vi "BucleWhile.vi"() -> ()   [LabVIEW 2020]
panel:
  in  "stop":bool
  in  "Tiempo apagado":dbl
  in  "Tiempo encendido":dbl
  out "Led":bool
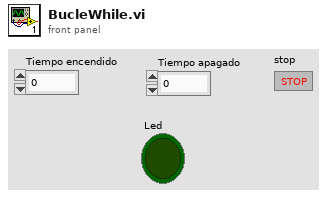
[diagram p1: front panel]
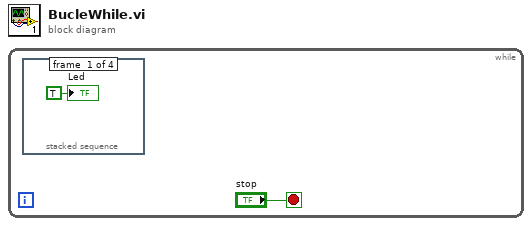
[diagram p0: block diagram]
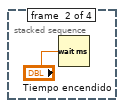
[diagram p2: hidden frame]
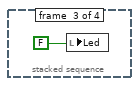
[diagram p3: hidden frame]
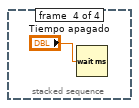
[diagram p4: hidden frame]
diagram:
  n1 = while {
    stop <- "stop" stop-if-true
    n2 = stacked-sequence {
      frame #0 {
        "Led" <- TRUE ("Led")
      }
      frame #1 {
        n3 = Wait (ms)(milliseconds to wait="Tiempo encendido") -> ()  [unwired: 1 out]
      }
      frame #2 {
        n4 = local write "Led"(FALSE ("Led")) -> ()
      }
      frame #3 {
        n5 = Wait (ms)(milliseconds to wait="Tiempo apagado") -> ()  [unwired: 1 out]
      }
    }
  }
